vi "Example 02d - Coroutines.vi"() -> ()   [LabVIEW 2020]
uses:
  Lua for LabVIEW/Lua/Lua.lvclass
panel:
  out "» Stack Dump 4":string[](array[string])
  out "» Stack Dump 3":string[](array[string])
  out "» Stack Dump 2":string[](array[string])
  out "» Stack Dump":string[](array[string])
  out "yielded indicies":i64[](array[numeric])
  in  "count":i64=2
  out "error out":errorcluster
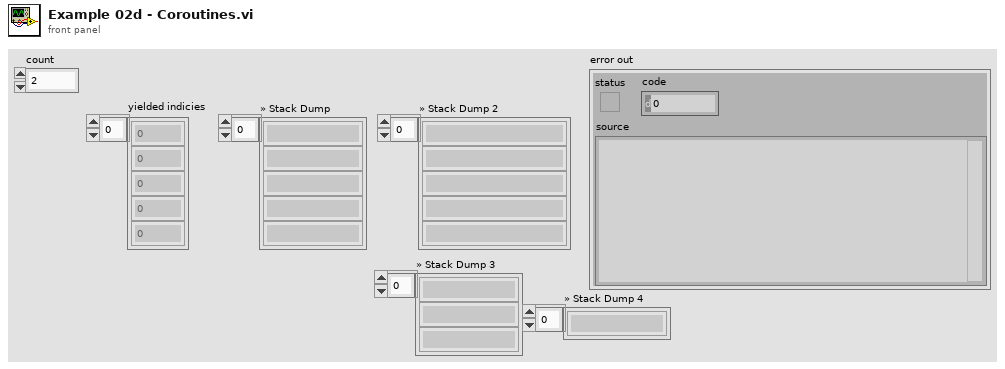
[diagram p1: front panel]
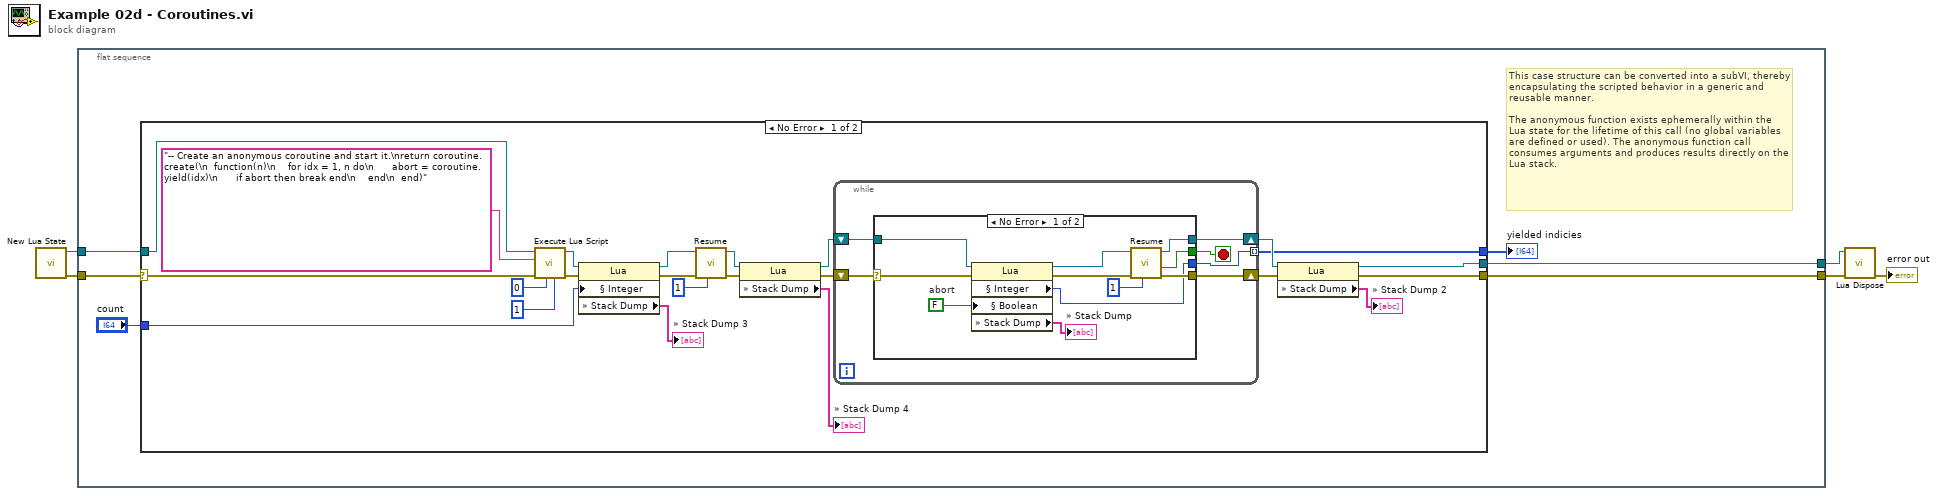
[diagram p0: block diagram]
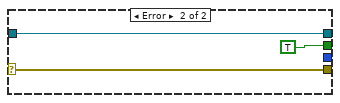
[diagram p2: hidden frame]
diagram:
  n1 = call "New Lua State.vi"() -> ("error out"=w4:errorcluster, "Lua out"=w5:refnum<data-value>)  [unwired: 10 in]
  n2 = flat-sequence {
    tunnel: w5 -> [w9]
    tunnel: w4 -> [w6]
    tunnel: [w11] -> w2
    tunnel: [w10] -> w1
    frame #0 {
      # "This case structure can be converted into a subVI, thereby encapsulating the scripted behavior in a generic and reusable manner.\n\nThe anonymous function exists ephemerally within the Lua state for the lifetime of this call (no global variables are defined or used). The anonymous function call consumes arguments and produces results directly on the Lua stack."
      n3 = case shown="No Error" w6 {
        selector: w6 -> [w23 w55]
        tunnel: [w28 w55] -> w11
        tunnel: [w29 w56] -> w10
        tunnel: w9 -> [w24 w56]
        tunnel: "count" -> [w34 _]
        tunnel: [w27 _] -> w7
        frame No Error {
          n4 = call "Execute Lua Script.vi"("nresults"=1, "nargs"=0, "error in (no error)"=w23, "lua script"="-- Create an anonymous coroutine and start it.\nreturn coroutine.create(\n  function(n)\n    for idx = 1, n do\n      abort = coroutine.yield(idx)\n      if abort then break end\n    end\n  end)", "Lua in"=w24) -> ("error out"=w19:errorcluster, "Lua out"=w22:refnum<data-value>)  [unwired: 5 in]
          n5 = property class="Lua"(reference=w22, error in=w19, "§ Integer"=w34) -> (reference out=w21:refnum<data-value>, error out=w20:errorcluster, "» Stack Dump"=→"» Stack Dump 3":string[])
          n6 = call "Resume.vi"("nargs"=1, "error in (no error)"=w20, "Lua in"=w21) -> ("error out"=w13:errorcluster, "Lua out"=w25:refnum<data-value>)  [unwired: 5 in, 2 out]
          n7 = property class="Lua"(reference=w25, error in=w13) -> (reference out=w15:refnum<data-value>, error out=w12:errorcluster, "» Stack Dump"=→"» Stack Dump 4":string[])
          n8 = while {
            shift-right: [w39] -> w30
            shift-left: w12 -> [w35]
            shift-right: [w40] -> w31
            shift-left: w15 -> [w36]
            tunnel: [w38] -> w27 mode=indexing
            stop <- w37 stop-if-true
            n9 = case shown="No Error" w35 {
              selector: w35 -> [w41 w54]
              tunnel: [w48 w52] -> w40
              tunnel: [w47 w54] -> w39
              tunnel: [w46 _] -> w38
              tunnel: [w45 TRUE] -> w37
              tunnel: w36 -> [w42 w52]
              frame No Error {
                w43 = FALSE  # abort
                n10 = property class="Lua"(reference=w42, error in=w41, "§ Boolean"=w43) -> (reference out=w51:refnum<data-value>, error out=w50:errorcluster, "§ Integer"=w46:i64, "» Stack Dump"=→"» Stack Dump":string[])
                n11 = call "Resume.vi"("nargs"=1, "error in (no error)"=w50, "Lua in"=w51) -> ("error out"=w47:errorcluster, "done?"=w45:bool, "Lua out"=w48:refnum<data-value>)  [unwired: 5 in, 1 out]
              }
              frame Error {
              }
            }
          }
          n12 = property class="Lua"(reference=w31, error in=w30) -> (reference out=w29:refnum<data-value>, error out=w28:errorcluster, "» Stack Dump"=→"» Stack Dump 2":string[])
        }
        frame Error {
        }
      }
      "yielded indicies" <- w7
    }
  }
  n13 = call "Lua Dispose.vi"("error in (no error)"=w2, "Disposable in"=w1) -> ("error out"=→"error out":errorcluster)  [unwired: 9 in]
